vi "main.vi"() -> ()   [LabVIEW 2018]
uses:
  <vilib>/Instr/_visa.llb/VISA Configure Serial Port (Instr).vi
panel:
  out "Serial flag":bool
  out "*(类型 *) &x 2":u32
  out "*(类型 *) &x":u32
  out "子字符串 3":string
  out "子字符串 2":string
  out "子字符串":string
  out "枚举":T1
  out "返回数":u32
  in  "baud rate":u64(ring) items=["9600"=9600, "14400"=14400, "115200"=115200]
  in  "write buffer":string
  in  "send":bool
  out "read buffer":string
  out "serial_state":bool
  in  "serial":refnum<visa-resource-name> caption="serial_select"
  in  "serial_open":bool
  in  "exit":bool
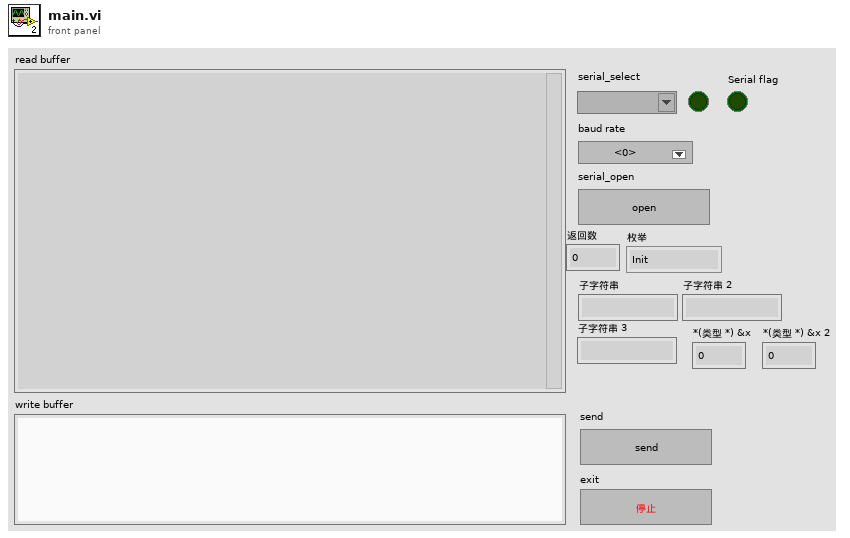
[diagram p1: front panel]
types:
  T1 = typedef "状态机.ctl" = enum16{"Init", "Send", "Wait", "GetData", "Deal", "Exit"}
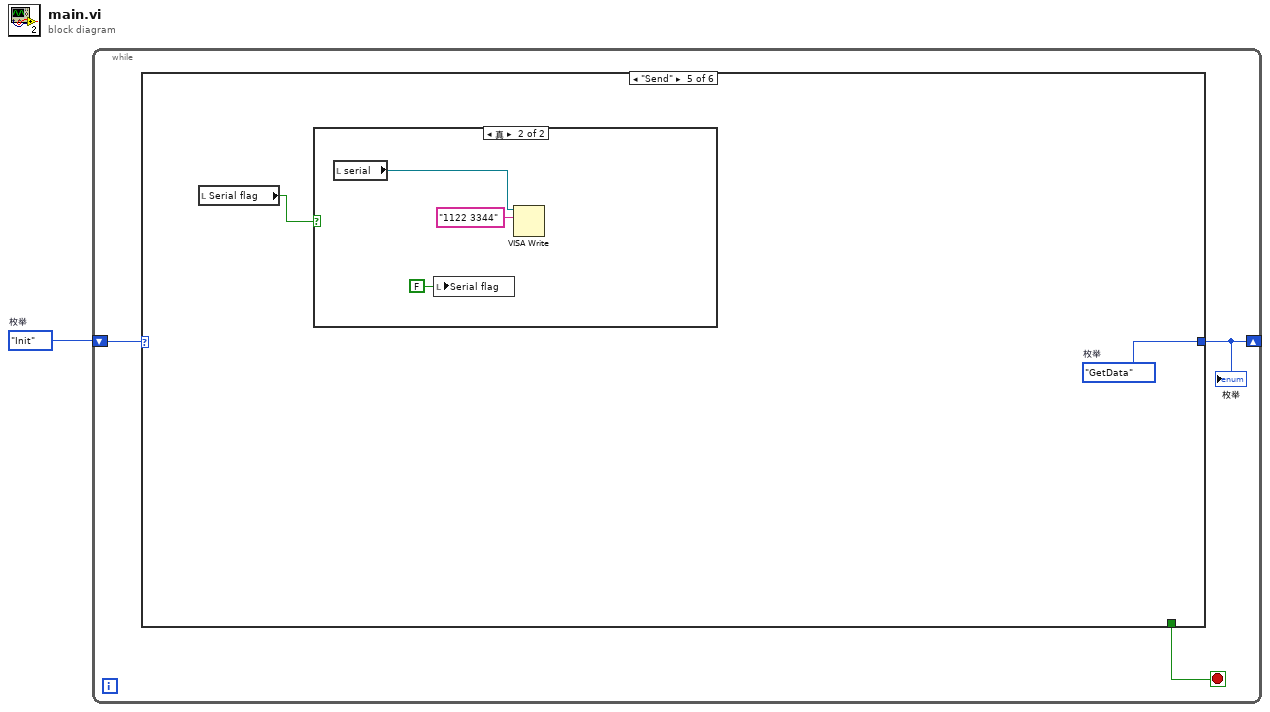
[diagram p0: block diagram]
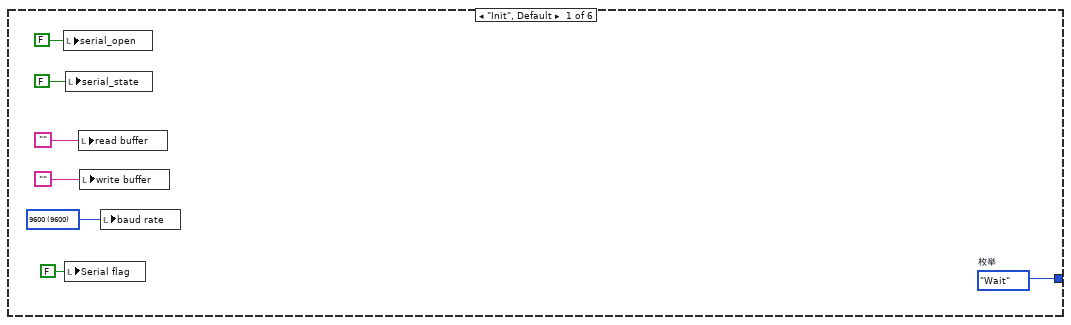
[diagram p2: hidden frame]
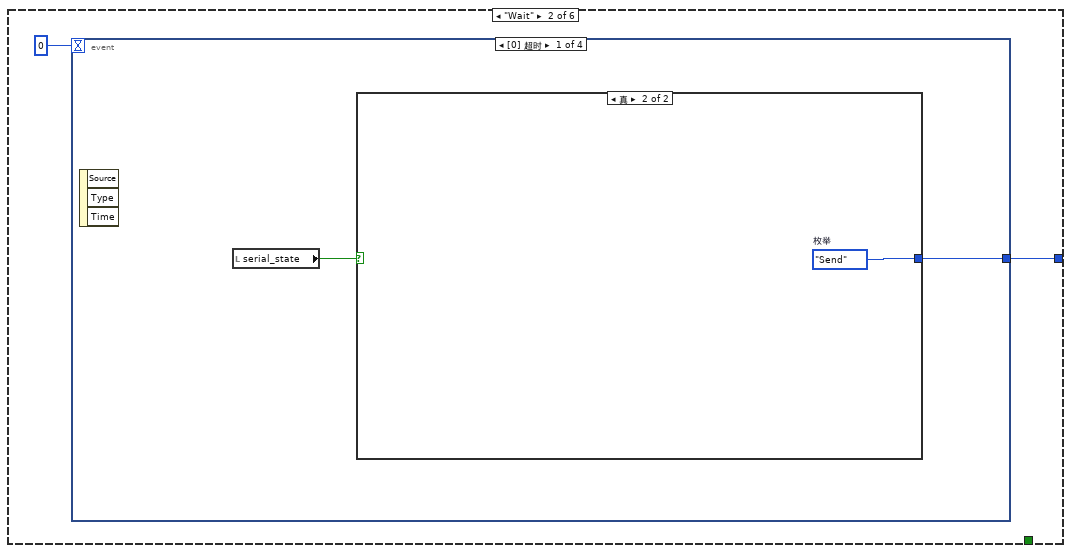
[diagram p3: hidden frame]
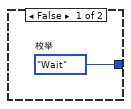
[diagram p4: hidden frame]
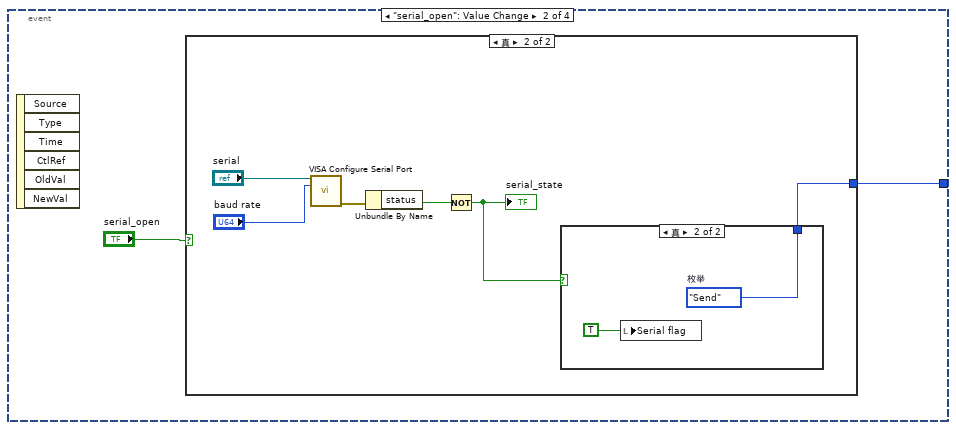
[diagram p5: hidden frame]
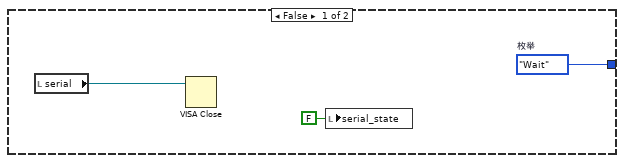
[diagram p6: hidden frame]
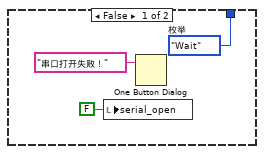
[diagram p7: hidden frame]
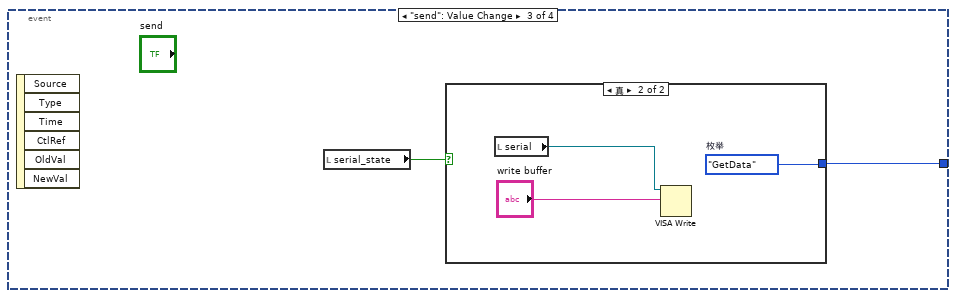
[diagram p8: hidden frame]
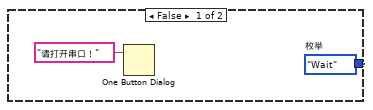
[diagram p9: hidden frame]
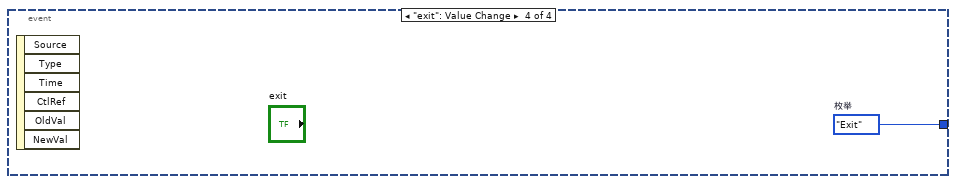
[diagram p10: hidden frame]
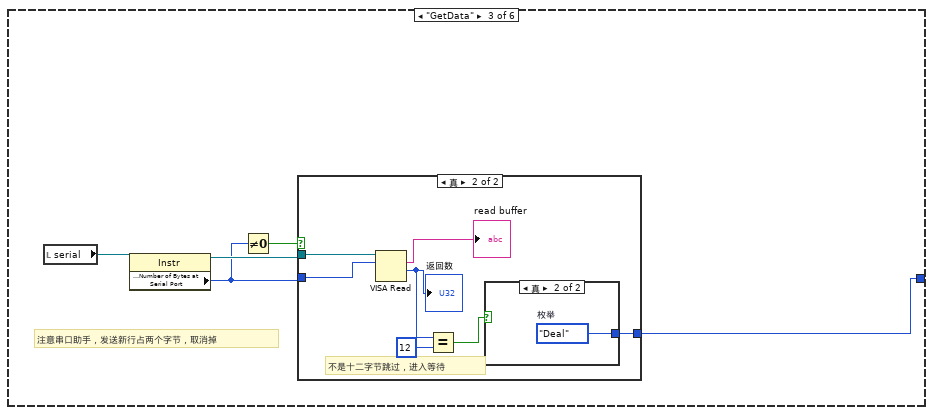
[diagram p11: hidden frame]
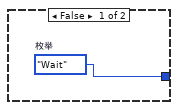
[diagram p12: hidden frame]
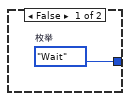
[diagram p13: hidden frame]
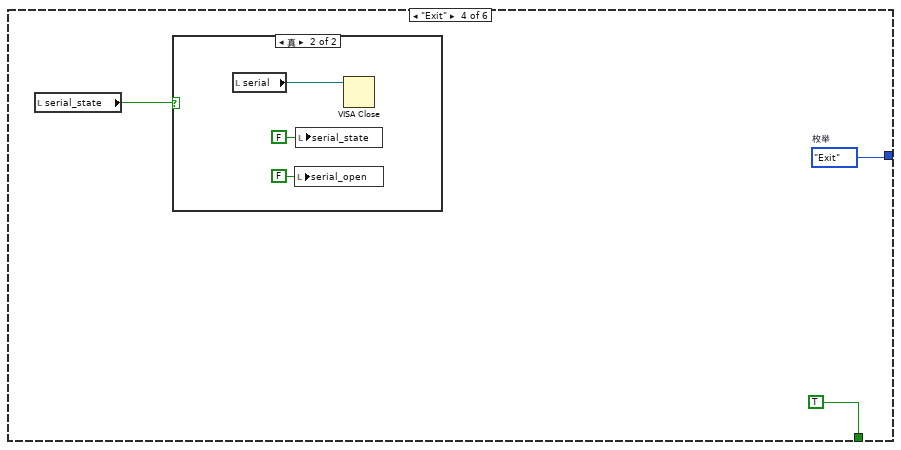
[diagram p14: hidden frame]
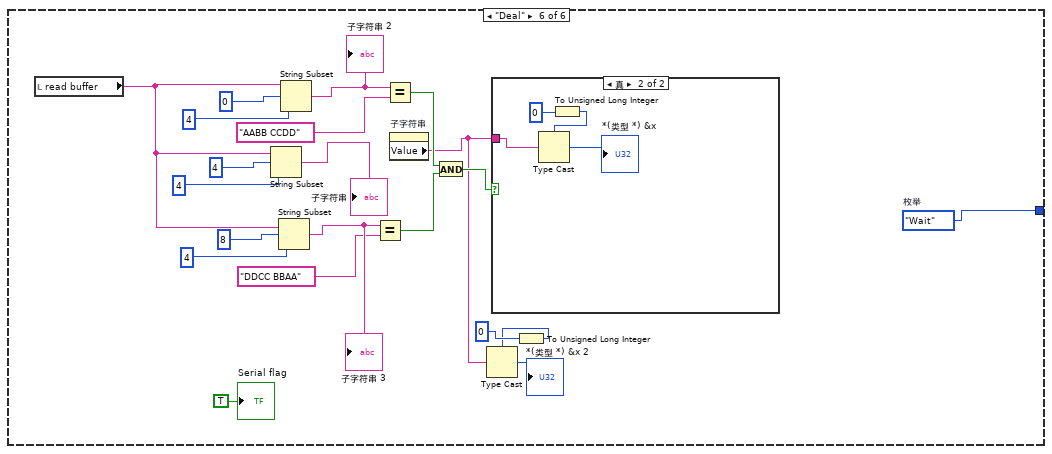
[diagram p17: hidden frame]
diagram:
  w1 = 状态机."Init"  # 枚举
  n1 = while {
    shift-right: [w3] -> _
    shift-left: w1 -> [w4]
    stop <- w2 stop-if-true
    n2 = case shown="\"Send\"" w4 {
      tunnel: [w9 w12 w42 w59 w63 w88] -> w3
      tunnel: [_ _ _ TRUE _ _] -> w2
      frame "Init", Default {
        w6 = u64 9600 items=["9600"=9600, "115200"=115200] ("baud rate")
        w9 = 状态机."Wait"  # 枚举
        n3 = local write "serial_open"(FALSE ("serial_open")) -> ()
        n4 = local write "Serial flag"(FALSE ("Serial flag")) -> ()
        n5 = local write "serial_state"(FALSE ("serial_state")) -> ()
        n6 = local write "read buffer"("") -> ()
        n7 = local write "write buffer"("") -> ()
        n8 = local write "baud rate"(w6) -> ()
      }
      frame "Wait" {
        n9 = event shown="[0] 超时" {
          selector: _ -> [_ _ _ _]
          dyn-events: _ -> [_ _ _ _]
          timeout: 0 -> [_ _ _ _]
          tunnel: [w14 w18 w34 w41] -> w12
          event Timeout {
            n10 = event-data() -> ()  [unwired: 1 in, 3 out]
            n11 = local read "serial_state"() -> (w15:bool)
            n12 = case shown="真" w15 {
              tunnel: [w16 w17] -> w14
              frame False {
                w16 = 状态机."Wait"  # 枚举
              }
              frame True {
                w17 = 状态机."Send"  # 枚举
              }
            }
          }
          event "serial_open": Value Change {
            n13 = event-data() -> ()  [unwired: 1 in, 6 out]
            n14 = case shown="真" "serial_open" {
              tunnel: [w20 w24] -> w18
              frame False {
                w20 = 状态机."Wait"  # 枚举
                n15 = local read "serial"() -> (w22:refnum<visa-resource-name>)
                n16 = VISA Close(VISA resource name=w22) -> ()  [unwired: 1 in, 1 out]
                n17 = local write "serial_state"(FALSE ("serial_state")) -> ()
              }
              frame True {
                n18 = call-poly "VISA Configure Serial Port"("VISA resource name"="serial", "baud rate (9600)"="baud rate") -> ("error out"=w27:errorcluster)  [unwired: 12 in, 1 out]
                n19 = Unbundle By Name(w27) -> ("status"=w26:bool)
                n20 = Not(x=w26) -> (.not. x?=w25:bool)
                "serial_state" <- w25
                n21 = case shown="真" w25 {
                  tunnel: [w29 w33] -> w24
                  frame False {
                    w29 = 状态机."Wait"  # 枚举
                    n22 = local write "serial_open"(FALSE ("serial_open")) -> ()
                    n23 = One Button Dialog(message="串口打开失败！" ("消息")) -> ()  [unwired: 1 in, 1 out]
                  }
                  frame True {
                    w33 = 状态机."Send"  # 枚举
                    n24 = local write "Serial flag"(TRUE ("Serial flag")) -> ()
                  }
                }
              }
            }
          }
          event "send": Value Change {
            n25 = event-data() -> ()  [unwired: 1 in, 6 out]
            n26 = local read "serial_state"() -> (w35:bool)
            n27 = case shown="真" w35 {
              tunnel: [w36 w38] -> w34
              frame False {
                w36 = 状态机."Wait"  # 枚举
                n28 = One Button Dialog(message="请打开串口！" ("消息")) -> ()  [unwired: 1 in, 1 out]
              }
              frame True {
                w38 = 状态机."GetData"  # 枚举
                n29 = local read "serial"() -> (w39:refnum<visa-resource-name>)
                n30 = VISA Write(VISA resource name=w39, write buffer="write buffer") -> ()  [unwired: 1 in, 3 out]
              }
            }
          }
          event "exit": Value Change {
            w41 = 状态机."Exit"  # 枚举
            n31 = event-data() -> ()  [unwired: 1 in, 6 out]
          }
        }
      }
      frame "GetData" {
        # "注意串口助手，发送新行占两个字节，取消掉"
        n32 = local read "serial"() -> (w43:refnum<visa-resource-name>)
        n33 = property class="Instr"(reference=w43) -> (reference out=w46:refnum<visa-resource-name>, "Serial Settings:Number of Bytes at Serial Port"=w44:u32)  [unwired: 1 in, 1 out]
        n34 = Not Equal To 0?(x=w44) -> (x != 0?=w45:bool)
        n35 = case shown="真" w45 {
          tunnel: w46 -> [_ w54]
          tunnel: w44 -> [_ w53]
          tunnel: [w47 w48] -> w42
          frame False {
            w47 = 状态机."Wait"  # 枚举
          }
          frame True {
            # "不是十二字节跳过，进入等待"
            n36 = VISA Read(VISA resource name=w54, byte count=w53) -> (read buffer=→"read buffer":string, return count=w51:u32)  [unwired: 1 in, 2 out]
            "返回数" <- w51
            n37 = Equal?(x=w51, y=u32 12) -> (x = y?=w49:bool)
            n38 = case shown="真" w49 {
              tunnel: [w55 w56] -> w48
              frame False {
                w55 = 状态机."Wait"  # 枚举
              }
              frame True {
                w56 = 状态机."Deal"  # 枚举
              }
            }
          }
        }
      }
      frame "Exit" {
        w59 = 状态机."Exit"  # 枚举
        n39 = local read "serial_state"() -> (w57:bool)
        n40 = case shown="真" w57 {
          frame False {
          }
          frame True {
            n41 = local read "serial"() -> (w62:refnum<visa-resource-name>)
            n42 = local write "serial_open"(FALSE ("serial_state")) -> ()
            n43 = local write "serial_state"(FALSE ("serial_state")) -> ()
            n44 = VISA Close(VISA resource name=w62) -> ()  [unwired: 1 in, 1 out]
          }
        }
      }
      frame "Send" {
        w63 = 状态机."GetData"  # 枚举
        n45 = local read "Serial flag"() -> (w64:bool)
        n46 = case shown="真" w64 {
          frame False {
          }
          frame True {
            n47 = local read "serial"() -> (w66:refnum<visa-resource-name>)
            n48 = local write "Serial flag"(FALSE ("Serial flag")) -> ()
            n49 = VISA Write(VISA resource name=w66, write buffer="1122 3344" ("写入缓冲区")) -> ()  [unwired: 1 in, 3 out]
          }
        }
      }
      frame "Deal" {
        w88 = 状态机."Wait"  # 枚举
        n50 = local read "read buffer"() -> (w81:string)
        n51 = String Subset(string=w81, offset (0)=4 ("偏移量(0)"), length (rest)=4 ("长度（剩余）")) -> (substring=→"子字符串":string)
        n52 = String Subset(string=w81, offset (0)=8 ("偏移量(0)"), length (rest)=4 ("长度（剩余）")) -> (substring=w79:string)
        "子字符串 3" <- w79
        n53 = String Subset(string=w81, offset (0)=0 ("偏移量(0)"), length (rest)=4 ("长度（剩余）")) -> (substring=w80:string)
        "子字符串 2" <- w80
        n54 = Equal?(x=w79, y="DDCC BBAA") -> (x = y?=w75:bool)
        n55 = Equal?(x=w80, y="AABB CCDD") -> (x = y?=w76:bool)
        n56 = property on="子字符串" class="Str"() -> ("Value"=w69:string)  [unwired: 2 in, 2 out]
        n57 = And(x=w76, y=w75) -> (x .and. y?=w74:bool)
        n58 = case shown="真" w74 {
          tunnel: w69 -> [_ w92]
          frame False {
          }
          frame True {
            n59 = To Unsigned Long Integer(number=0) -> (unsigned 32bit integer=w90:u32)
            n60 = Type Cast(type=w90, x=w92) -> (*(type *) &x=→"*(类型 *) &x":u32)
          }
        }
        n61 = To Unsigned Long Integer(number=0) -> (unsigned 32bit integer=w71:u32)
        n62 = Type Cast(type=w71, x=w69) -> (*(type *) &x=→"*(类型 *) &x 2":u32)
        "Serial flag" <- TRUE ("Serial flag")
      }
    }
    "枚举" <- w3
  }
